vi "Get Controller Rate.vi"(8 "error in (no error)":errorcluster, 11 "Device Reference In":T1=18446744073709551615 format="%.0x") -> (0 "error out":errorcluster, 1 "Rate in Hz":dbl, 2 "System dt in uS":u32, 3 "Device Reference dup":T1=18446744073709551615 format="%.0x")   [LabVIEW 2011, in "PXIe-433x Custom Device.lvlib"]
uses:
  PXIe-433x Custom Device.lvlib
  <vilib>/NI Veristand/Custom Device API/Custom Device Item Ref.ctl
  <vilib>/NI Veristand/Custom Device Tools/Custom Device Utility Library/Custom Device Utility Library.lvlib
  <vilib>/NI Veristand/Custom Device API/Custom Device API.lvlib
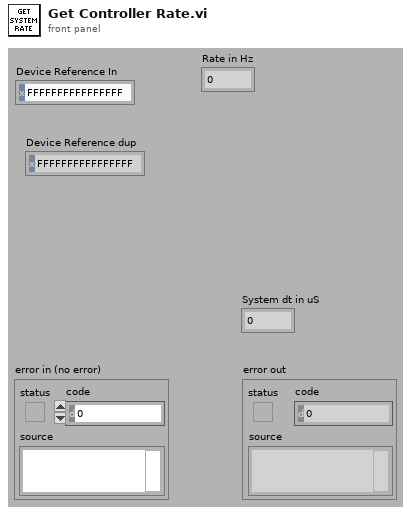
[diagram p1: front panel]
types:
  T1 = typedef "Custom Device API.lvlib/Custom Device Item Ref.ctl" = u64
  T2 = typedef "Custom Device API.lvlib/Custom Device Channel.ctl" = cluster{"Type":T3, "Units":string, "Default Value":dbl, "Faultable":bool, "Scalable":bool}
  T3 = typedef "Custom Device API.lvlib/Custom Device Channel Type.ctl" = enum16{"Input", "Output"}
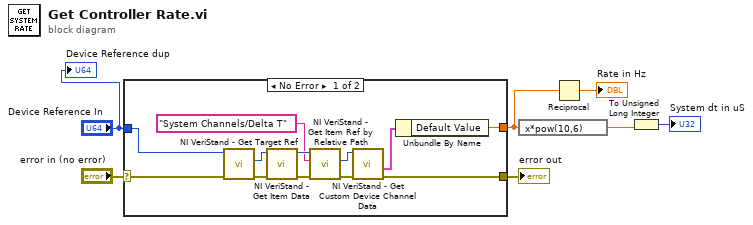
[diagram p0: block diagram]
diagram:
  n1 = case shown="No Error" "error in (no error)" {
    selector: "error in (no error)" -> [w8 w20]
    tunnel: [w11 w20] -> w7
    tunnel: "Device Reference In" -> [w9 _]
    tunnel: [w10 _] -> w3
    frame No Error {
      n2 = call <vilib>:"NI VeriStand - Get Target Ref.vi"("error in"=w8, "Item Ref in"=w9) -> ("error out"=w18:errorcluster, "Target Ref"=w19:T1)  [unwired: 8 out]
      n3 = call <vilib>:"NI VeriStand - Get Item Data.vi"("error in (no error)"=w18, "Item Ref in"=w19) -> ("error out"=w16:errorcluster, "Item Ref out"=w17:T1)  [unwired: 8 out]
      n4 = call <vilib>:"NI VeriStand - Get Item Ref by Relative Path.vi"("error in"=w16, "Relative Item Path"="System Channels/Delta T", "Section Ref in"=w17) -> ("error out"=w13:errorcluster, "Item Ref"=w14:T1)  [unwired: 7 out]
      n5 = call <vilib>:"NI VeriStand - Get Custom Device Channel Data.vi"("error in (no error)"=w13, "Channel Ref in"=w14) -> ("error out"=w11:errorcluster, "Channel"=w12:T2)  [unwired: 8 out]
      n6 = Unbundle By Name(w12) -> ("Default Value"=w10:dbl)
    }
    frame Error {
    }
  }
  "error out" <- w7
  n7 = expression code="x*pow(10,6)"(w3) -> (w4:dbl)
  n8 = Reciprocal(x=w3) -> (1/x=→"Rate in Hz":dbl)
  n9 = To Unsigned Long Integer(number=w4) -> (unsigned 32bit integer=→"System dt in uS":u32)
  "Device Reference dup" <- "Device Reference In"
